vi "Get map dimensions.vi"(0 "all rows":string[][](array[string])) -> (1 "Step":dbl, 2 "Y0":dbl, 3 "X0":dbl)   [LabVIEW 2009]
uses:
  <vilib>/Analysis/NI_AALPro.lvlib
  <vilib>/regexp/Match Regular Expression.xnode
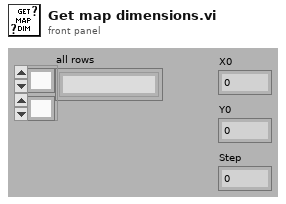
[diagram p1: front panel]
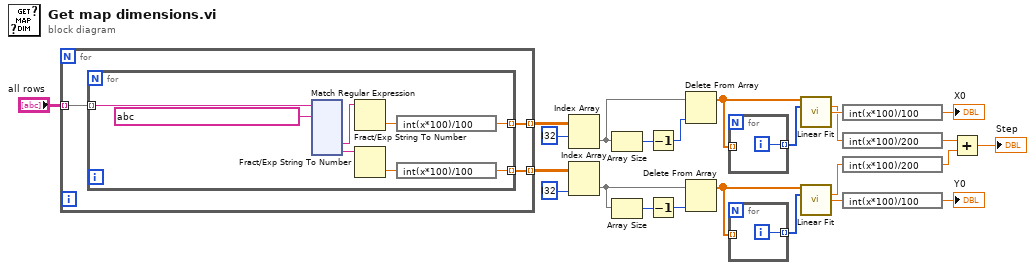
[diagram p0: block diagram]
diagram:
  n1 = for {
    tunnel: "all rows" -> [w27] mode=indexing
    tunnel: [w26] -> w6 mode=indexing
    tunnel: [w25] -> w4 mode=indexing
    n2 = for {
      tunnel: w27 -> [w35] mode=indexing
      tunnel: [w31] -> w26 mode=indexing
      tunnel: [w28] -> w25 mode=indexing
      n3 = xnode "Match Regular Expression"("input string"=w35, "regular expression"=string ?) -> ("submatch 1"=w33:string, "submatch 2"=w32:string)  [unwired: 4 in, 5 out]
      n4 = Fract/Exp String To Number(string=w33) -> (number=w30:dbl)  [unwired: 3 in, 1 out]
      n5 = Fract/Exp String To Number(string=w32) -> (number=w29:dbl)  [unwired: 3 in, 1 out]
      n6 = expression code="int(x*100)/100"(w30) -> (w31:dbl)
      n7 = expression code="int(x*100)/100"(w29) -> (w28:dbl)
    }
  }
  n8 = Index Array(array=w6, index (row)=i32 ?) -> (element=w17:dbl[])  [unwired: 1 in]
  n9 = Index Array(array=w4, index (col)=i32 ? ("index (row)")) -> (element=w7:dbl[])  [unwired: 1 in]
  n10 = Array Size(array=w17) -> (size(s)=w18:i32)
  n11 = Array Size(array=w7) -> (size(s)=w8:i32)
  n12 = Decrement(x=w18) -> (x-1=w19:i32)
  n13 = Decrement(x=w8) -> (x-1=w9:i32)
  n14 = Delete From Array(array=w17, index=w19) -> (array with subset deleted=w24:dbl[])  [unwired: 1 in, 1 out]
  n15 = Delete From Array(array=w7, index=w9) -> (array with subset deleted=w14:dbl[])  [unwired: 1 in, 1 out]
  n16 = for {
    tunnel: w24 -> [_] mode=indexing
    tunnel: [w150] -> w23 mode=indexing
    i -> [w150]
  }
  n17 = for {
    tunnel: w14 -> [_] mode=indexing
    tunnel: [w151] -> w13 mode=indexing
    i -> [w151]
  }
  n18 = call <vilib>:"Linear Fit.vi"("Y"=w24, "X"=w23) -> ("slope"=w20:dbl, "intercept"=w21:dbl)  [unwired: 9 in, 3 out]
  n19 = call <vilib>:"Linear Fit.vi"("Y"=w14, "X"=w13) -> ("slope"=w10:dbl, "intercept"=w11:dbl)  [unwired: 9 in, 3 out]
  n20 = expression code="int(x*100)/100"(w21) -> (→"X0":dbl)
  n21 = expression code="int(x*100)/200"(w20) -> (w3:dbl)
  n22 = expression code="int(x*100)/200"(w10) -> (w2:dbl)
  n23 = expression code="int(x*100)/100"(w11) -> (→"Y0":dbl)
  n24 = Add(x=w3, y=w2) -> (x+y=→"Step":dbl)
